vi "Read Parameter.vi"(8 "error in (no error)":errorcluster, 11 "SqlMapper in":refnum<class "SqlMapper.lvclass">) -> (0 "error out":errorcluster, 2 "DynamicParameters out":refnum<class "DynamicParameters.lvclass">, 3 "SqlMapper out":refnum<class "SqlMapper.lvclass">)   [LabVIEW 2020, in "ORM.lvlib" / "SqlMapper.lvclass"]
uses:
  SqlMapper.lvclass
  DynamicParameters/DynamicParameters.lvclass
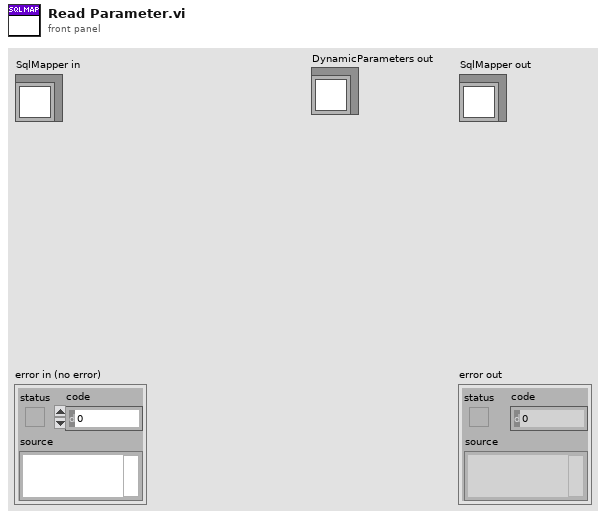
[diagram p1: front panel]
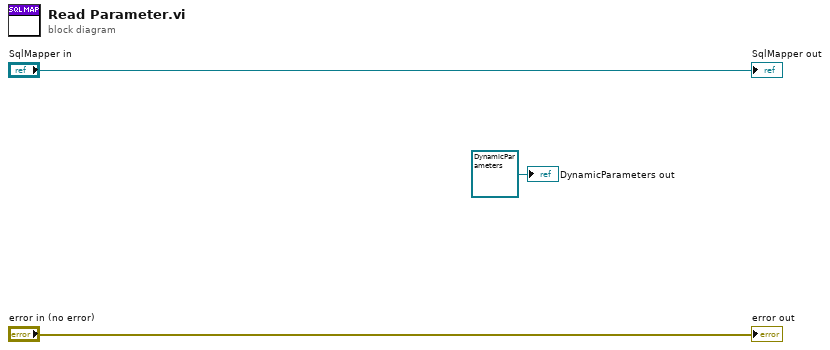
[diagram p0: block diagram]
diagram:
  "error out" <- "error in (no error)"
  "SqlMapper out" <- "SqlMapper in"
  "DynamicParameters out" <- refnum<class "DynamicParameters.lvclass"> refnum ("DynamicParameters out")
